vi "Join_8BitData.vi"(0 "hi":u8 format="%.0x", 2 "lo":u8 format="%.0x") -> (15 "hi.lo(8bits)":u8 format="%.0x")   [LabVIEW 2023, in "HardwareAbstractionLayer_LVOOP.lvlib" / "CAN Application Protocols Lib.lvlib" / "STP Protocol.lvclass"]
uses:
  STP Protocol.lvclass
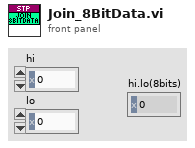
[diagram p1: front panel]
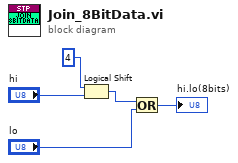
[diagram p0: block diagram]
diagram:
  n1 = Logical Shift(y=u8 4 ("unsigned 8bit integer"), x="hi") -> (x << y=w3:u8)
  n2 = Or(x=w3, y="lo") -> (x .or. y?=→"hi.lo(8bits)":u8)
